vi "Auto Elevator Mode.vi"(0 "Elevator Command":T3={"Command"=enum."Idle", "Manual Motor Out"=0.0, "Manual Eject Piston"=FALSE, "Mode"=enum."Manual", "Override Limits"=FALSE, "Manual Stabilizer"=FALSE, "Manual Finger"=FALSE, "Store Trashcan?"=FALSE, "Hold Low?"=FALSE, "Idle Mode"=enum."Load Can", "HP Load"=FALSE}, 2 "reinitialize? (F)":bool, 5 "Current Position":dbl, 9 "Object In?":bool, 11 "Finger Height":dbl) -> (4 "Auto Elevator Indicators":T1, 6 "output":dbl, 8 "Finger Out":bool, 10 "Stabilizer Out":bool, 14 "Finger at bottom":bool, 15 "Eject Out":bool)   [LabVIEW 2014]
uses:
  Elevator Control Command.ctl
  Elevator Command.ctl
  Common Code/Elevator Mode.ctl
  Common Code/Elevator Idle Mode.ctl
  Common Code/Auto Elevator Indicators.ctl
  Common Code/Elevator State.ctl
  Elevator Sensors.ctl
  Robot Global Data.vi
  <vilib>/addons/control/pid/pid.llb/PID (DBL).vi
  <vilib>/addons/control/pid/NI_PID_pid.lvlib
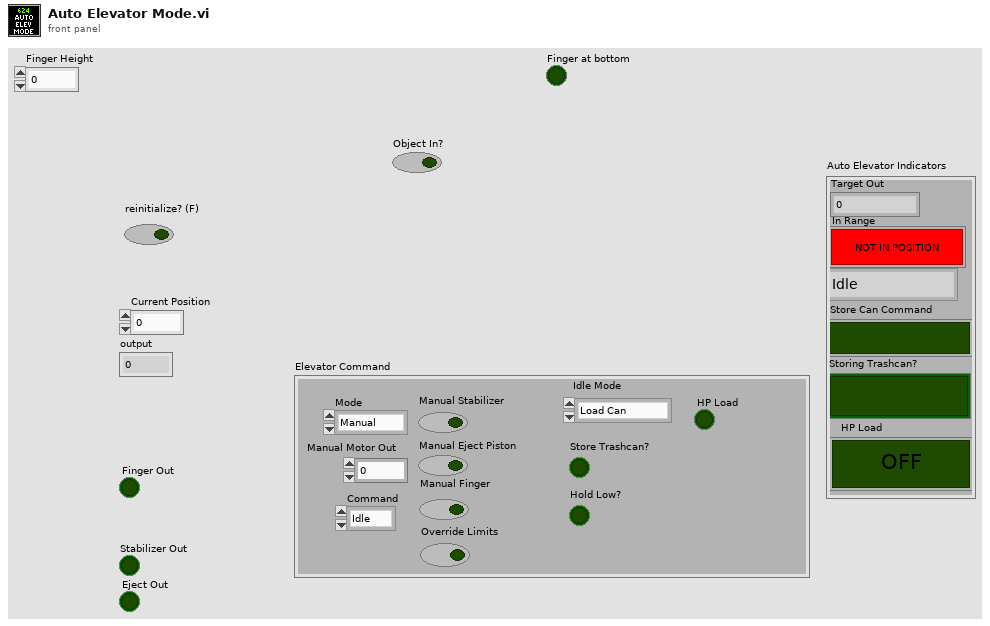
[diagram p1: front panel]
types:
  T1 = typedef "Auto Elevator Indicators.ctl" = cluster{"Target Out":dbl, "Storing Trashcan?":bool, "State":T2, "In Range":bool, "Store Can Command":bool, "HP Load":bool}
  T2 = typedef "Elevator State.ctl" = enum16{"Idle", "Goto Load Position", "Wait for Load", "Load Drop", "Load Lift", "Drop Stack", "Goto Eject Position", "Eject ", "Raise Trashcan", "Open Stabilizer", "Untip Drop", "Untip Wait", "Untip Lift", "Abort Load", "HP Load Wait", "HP Load Drop", "HP Load Lift", "HP Load Abort", "Close Stabilizer", "HP Load Lift First Tote", "HP Load Drop First Tote", "HP Load Unfinish", "HP Drag Score", "HP Drag Finish Up", "HP Drag Finish Down", "HP Carry Finish Drop", "HP Carry Finish Lift", "HP Carry Score"}
  T3 = typedef "Elevator Control Command.ctl" = cluster{"Command":T4, "Manual Motor Out":dbl, "Manual Eject Piston":bool, "Mode":T5, "Override Limits":bool, "Manual Stabilizer":bool, "Manual Finger":bool, "Store Trashcan?":bool, "Hold Low?":bool, "Idle Mode":T6, "HP Load":bool}
  T4 = typedef "Elevator Command.ctl" = enum16{"Idle", "Load 1", "Load 2", "Load 3", "Drop Stack", "Eject Stack", "Untip Trashcan", "Load Trashcan", "HP Load", "HP Score"}
  T5 = typedef "Elevator Mode.ctl" = enum16{"Manual", "Safe", "Auto"}
  T6 = typedef "Elevator Idle Mode.ctl" = enum16{"Load 1", "Load 2", "Load 3", "Load Can", "Untip Can", "Step Load", "Drop Stack"}
  T7 = typedef "Elevator Status.ctl" = cluster{"Height":dbl, "Enc Value":dbl, "Limit Override":bool, "Mode":T5, "High IR":bool, "Motor Out":dbl, "Ping Detect":bool, "Auto Elevator Indicators":T1, "Master Current":dbl, "Slave Current":dbl, "High Current":bool, "Current Tripped":bool, "Top Limit":bool, "Bottom Limit":bool, "Eject Piston":bool, "Stabilizer":bool, "Finger":bool, "Finger Height":dbl, "Finger Raw":dbl, "Finger at Bottom":bool}
  T8 = typedef "Elevator Sensors.ctl" = cluster{"Object In?":bool, "Elevator in Position?":bool, "Current Position":dbl, "Abort Load":bool, "Finger Height":dbl, "Finger at bottom?":bool}
  T9 = typedef "Dashboard Control Data.ctl" = cluster{"Cam Exposure":dbl, "Go to angle":dbl, "Steer PID Gains":cluster{"proportional gain (Kc)":dbl, "integral time (Ti, min)":dbl, "derivative time (Td, min)":dbl}, "Steer PID output Range":cluster{"output high":dbl, "output low":dbl}, "Pressure m \nValue":dbl, "Pressure b \nValue":dbl, "Roller Command Cluster ":T10, "Elevator":T11, "Encoder Control":T13, "Auton Settings":cluster{"Drive Dist Window Size":dbl}, "Drivetrain Settings":T14}
  T10 = typedef "Roller Control.ctl" = cluster{"Intake Speed":dbl, "Turn In Speed":dbl, "Unload Speed":dbl, "Turn Out Speed":dbl, "Ping Align Tolerance":dbl, "Tote Range Threshold":dbl, "Right Pot 0":dbl, "Pot Threshold":dbl, "Left Pot 0":dbl, "Manual 0s?":bool, "Right Pot Scale":dbl, "Left Pot Scale":dbl, "0 wait time":i32, "Zero Pots":bool, "Min Elevator Height":dbl, "Eject Time":dbl, "Eject US Threshold":dbl, "Anti-Twitch Time":u32, "Ping Caring Threshold":dbl, "Pot Diff Threshold":dbl, "Pinch Sustain":u32, "Absorb Give Up Threshold":dbl, "Untip In Threshold":dbl, "Untip Grab Range":dbl, "Ultrasonic Hold Time":u32, "Landscape Absorb Time":u32, "Pot Use Wait Time":u32, "Can Turn Stop Range":dbl, "Ignore Pressure":bool, "HP Load Speed":dbl}
  T11 = typedef "Elevator DB Control.ctl" = cluster{"PID Output Range":cluster{"output high":dbl, "output low":dbl}, "PID gains":cluster{"proportional gain (Kc)":dbl, "integral time (Ti, min)":dbl, "derivative time (Td, min)":dbl}, "Height Tolerance":sgl, " Encoder Constant":dbl, "Safe Mode Max Speed":sgl, "Eject Time":sgl, "Zeroing Speed":sgl, "Presets":T12, "Ping Detect Threshold":sgl, "Trashcan Detect Threshold":sgl, "Zero Filter Time":dbl, "Stabilizer Open Time":dbl, "Zero Creep Speed":dbl, "Max Current":dbl, "Current Trip Time":dbl, "Abort Pitch":dbl, "Finger m":dbl, "Finger b":dbl, "Finger max ":dbl, "Finger Stabilizer":dbl, "Finger Store":dbl, "Finger Stop Store":dbl, "Stabilizer Close Time":dbl, "HP Finger Store":dbl, "HP Finger Stop Store":dbl, "Finger min":dbl}
  T12 = typedef "Elevator Presets.ctl" = cluster{"Pickup 2 w/ Tote":sgl, "Pickup 2 w/ Trashcan":sgl, "Pickup 3 w/ Tote":sgl, "Pickup 3 w/ Trashcan":sgl, "Bottom":sgl, "Pickup 1 w/ Tote":sgl, "Pickup Trashcan":sgl, "Pickup 1 w/ Trashcan":sgl, "Eject":sgl, "Hold Low":sgl, "Step add height":sgl, "Untip Lift":dbl, "Drop Stack":dbl, "HP Load Hold":dbl, "HP Load Drop":dbl, "HP Load Finger":dbl, "HP Load Hold Can":dbl, "Store can max":dbl, "HP Drag Score":dbl, "HP Store can max":dbl, "HP Drag Finish":dbl, "HP Carry min":dbl, "HP Finger Anti-Crash":dbl, "Finger trashcan avoid":dbl}
  T13 = typedef "Encoder Control.ctl" = cluster{"Left Tick Constant":dbl, "Right Tick Constant":dbl, "Center Tick Constant":dbl, "Reset?":bool, "Y Dist":cluster{"PID gains":cluster{"proportional gain (Kc)":dbl, "integral time (Ti, min)":dbl, "derivative time (Td, min)":dbl}}, "X Dist":cluster{"PID gains":cluster{"proportional gain (Kc)":dbl, "integral time (Ti, min)":dbl, "derivative time (Td, min)":dbl}}, "Y Stop Thresh":dbl, "Y Stop Speed":dbl, "X Stop Thresh":dbl, "X Stop Speed":dbl}
  T14 = typedef "Drivetrain Settings.ctl" = cluster{"Gyro Tolerance":sgl, "Strafe Correct max steer":sgl, "Strafe Timer Wait":sgl, "Throttle Ramp (ms)":sgl, "Strafe Ramp (ms)":sgl, "Angular rate compensation":bool, "Throttle to Rate Scale":sgl, "Rate compensation gain":sgl, "Creep Steer":sgl, "Creep Throttle":sgl}
  T15 = typedef "IMU Data.ctl" = cluster{"Pitch":sgl, "Roll":sgl, "Yaw":sgl, "Data Valid?":bool, "Temp":sgl, "MOVING":bool, "NAVX_CAL_STATUS":T16, "NAVX_OP_STATUS":T17, "YAW_STABLE":bool, "Accel X":sgl, "Accel Y":sgl, "Accel Z":sgl, "Accel Magnitude":sgl, "Pitch Rate":sgl, "Roll Rate":sgl, "Yaw Rate":sgl}
  T16 = typedef "navX-MXP IMU.lvlib/navX NAVX_CAL_STATUS.ctl" = u8
  T17 = typedef "navX-MXP IMU.lvlib/navX NAVX_OP_STATUS.ctl" = u8
  T18 = typedef "Elevator Actuators.ctl" = cluster{"Ejector Piston":bool, "Finger":bool, "Stabilizer":bool, "Position Out":dbl}
  T19 = cluster{"proportional gain (Kc)":dbl, "integral time (Ti, min)":dbl, "derivative time (Td, min)":dbl}
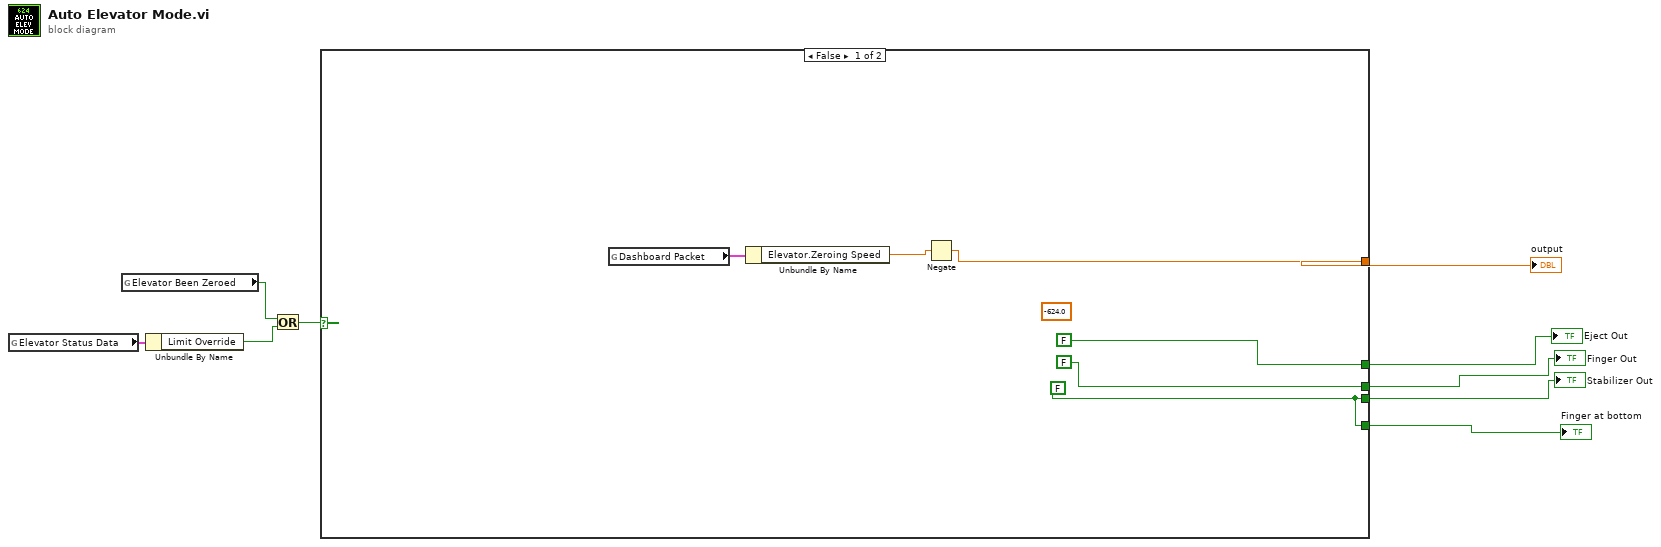
[diagram p0: block diagram]
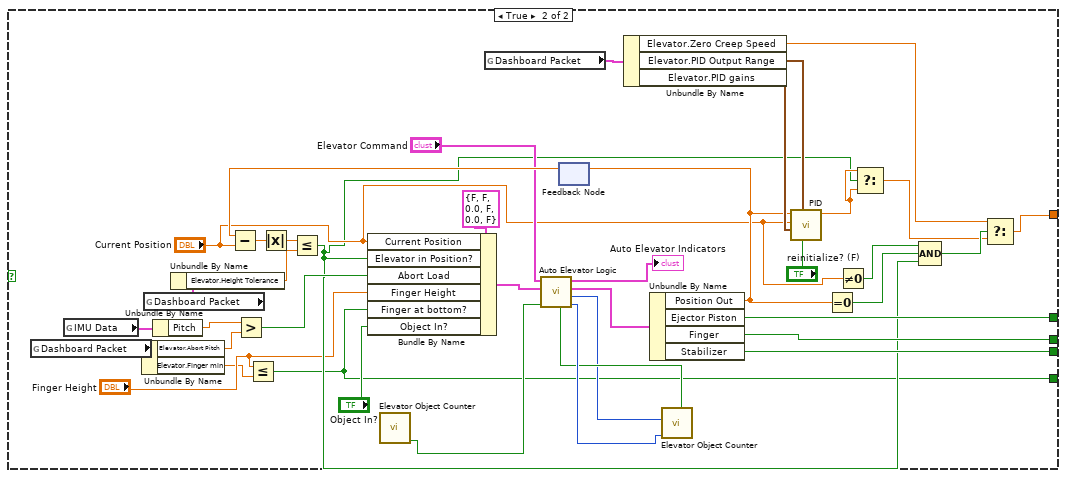
[diagram p2: hidden frame]
diagram:
  n1 = global read "Robot Global Data.vi" "Elevator Status Data"() -> (w5:T7)
  n2 = global read "Robot Global Data.vi" "Elevator Been Zeroed"() -> (w4:bool)
  n3 = Unbundle By Name(w5) -> ("Limit Override"=w3:bool)
  n4 = Or(x=w4, y=w3) -> (x .or. y?=w2:bool)
  n5 = case shown="False" w2 {
    tunnel: [w11 w33] -> w9
    tunnel: [FALSE ("Ejector Piston") w41] -> w8
    tunnel: [FALSE ("Finger") w40] -> w7
    tunnel: [w10 w39] -> w6
    tunnel: [w10 w16] -> w1
    frame False {
      (unwired) -624.0 ("Position Out")
      w10 = FALSE ("Stabilizer")
      n6 = global read "Robot Global Data.vi" "Dashboard Packet"() -> (w13:T9)
      n7 = Unbundle By Name(w13) -> ("Elevator.Zeroing Speed"=w12:sgl)
      n8 = Negate(x=w12) -> (-x=w11:sgl)
    }
    frame True {
      n9 = global read "Robot Global Data.vi" "Dashboard Packet"() -> (w28:T9)
      n10 = global read "Robot Global Data.vi" "IMU Data"() -> (w30:T15)
      n11 = Unbundle By Name(w28) -> ("Elevator.Abort Pitch"=w27:dbl, "Elevator.Finger min"=w17:dbl)
      n12 = global read "Robot Global Data.vi" "Dashboard Packet"() -> (w38:T9)
      n13 = Unbundle By Name(w30) -> ("Pitch"=w29:sgl)
      n14 = Unbundle By Name(w38) -> ("Elevator.Height Tolerance"=w51:sgl)
      n15 = Greater?(x=w29, y=w27) -> (0:w26:bool)
      n16 = Less Or Equal?(x="Finger Height", y=w17) -> (x <= y?=w16:bool)
      n17 = call "Elevator Object Counter.vi"() -> ("Have Trashcan"=w45:bool)  [unwired: 10 in, 1 out]
      n18 = global read "Robot Global Data.vi" "Dashboard Packet"() -> (w48:T9)
      n19 = feedback #1() -> (w52:dbl)  [unwired: 1 in]
      n20 = Subtract(x=w52, y="Current Position") -> (x-y=w54:dbl)
      n21 = Absolute Value(x=w54) -> (abs(x)=w55:dbl)
      n22 = Less Or Equal?(x=w55, y=w51) -> (x <= y?=w21:bool)
      n23 = Bundle By Name(cluster=T8 {"Object In?"=FALSE, "Elevator in Position?"=FALSE, "Current Position"=0.0, "Abort Load"=FALSE, "Finger Height"=0.0, "Finger at bottom?"=FALSE} ("Elevator Sensors In"), "Current Position"="Current Position", "Elevator in Position?"=w21, "Abort Load"=w26, "Finger Height"="Finger Height", "Finger at bottom?"=w16, "Object In?"="Object In?") -> (w49:T8)
      n24 = call "Auto Elevator Logic.vi"("Has Trashcan?"=w45, "Elevator Sensors In"=w49, "Command"="Elevator Command") -> ("Trashcan Delta"=w44:i32, "Tote Delta"=w19:i16, "Elevator Actuators Out"=w53:T18, "Auto Elevator Indicators"=→"Auto Elevator Indicators":T1, "Clear Stack Count"=w42:bool)  [unwired: 4 in]
      n25 = Unbundle By Name(w48) -> ("Elevator.Zero Creep Speed"=w32:dbl, "Elevator.PID Output Range"=w47:cluster{"output high":dbl, "output low":dbl}, "Elevator.PID gains"=w46:T19)
      n26 = Unbundle By Name(w53) -> ("Position Out"=w35:dbl, "Ejector Piston"=w41:bool, "Finger"=w40:bool, "Stabilizer"=w39:bool)
      n27 = feedback-in #1(w35) -> ()
      n28 = call "Elevator Object Counter.vi"("Clear Stack?"=w42, "Trashcan Delta"=w44, "Tote Delta"=w19) -> ()  [unwired: 7 in, 2 out]
      n29 = call-poly <vilib>:"PID.vi"("reinitialize? (F)"="reinitialize? (F)", "output range"=w47, "PID gains"=w46, "process variable"="Current Position", "setpoint"=w35) -> ("output"=w24:dbl)  [unwired: 5 in, 1 out]
      n30 = Equal To 0?(x=w35) -> (x = 0?=w22:bool)
      n31 = Not Equal To 0?(x="Current Position") -> (x != 0?=w23:bool)
      n32 = Select(t=w24, s=w21, f=w24) -> (s? t:f=w25:dbl)
      n33 = Compound Arithmetic op=AND(w23, w22, w21) -> (w31:bool)
      n34 = Select(t=w32, s=w31, f=w25) -> (s? t:f=w33:dbl)
    }
  }
  "output" <- w9
  "Eject Out" <- w8
  "Finger Out" <- w7
  "Stabilizer Out" <- w6
  "Finger at bottom" <- w1
